vi "VI-Find Get Events Bottom.vi"(0 "VI in":refnum<vi>, 11 "error in (no error)":errorcluster) -> (4 "VI out":refnum<vi>, 6 "bundler":refnum<vi>, 10 "# of constants":i32, 13 "function pos":T1, 14 "constant pos":T1, 15 "error out":errorcluster)   [LabVIEW 2015]
uses:
  <vilib>/Utility/miscctls.llb/LVPointTypeDef.ctl
  <vilib>/Utility/traverseref.llb/TRef TravTarget.ctl
  <vilib>/Utility/traverseref.llb/VI Scripting - Traverse.lvlib
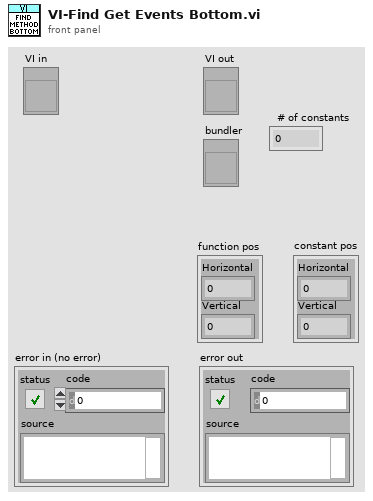
[diagram p1: front panel]
types:
  T1 = typedef "LVPointTypeDef.ctl" = cluster{"Horizontal":i16, "Vertical":i16}
  T2 = typedef "TRef TravTarget.ctl" = enum16{"FP", "BD", "Other"}
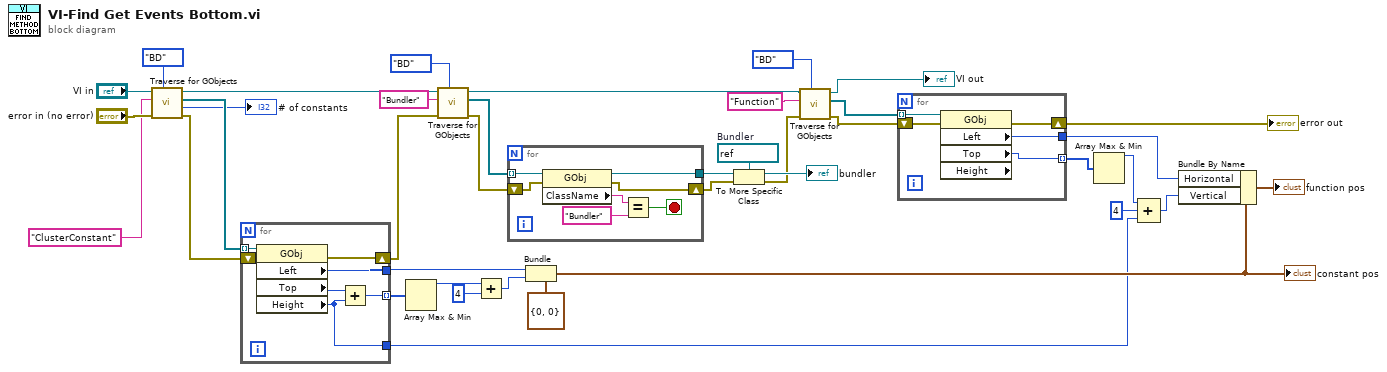
[diagram p0: block diagram]
diagram:
  w20 = refnum<vi> refnum  # Bundler
  n1 = call <vilib>:"Traverse for GObjects.vi"("Traverse Target"=TRef_TravTarget."BD", "error in (no error)"="error in (no error)", "Class Name"="ClusterConstant", "VI Refnum"="VI in") -> ("error out"=w28:errorcluster, "# of Refs"=→"# of constants":i32, "References"=w35:refnum<vi>[], "dup VI Refnum"=w27:refnum<vi>)  [unwired: 4 in]
  n2 = for {
    tunnel: w35 -> [w46] mode=indexing
    tunnel: [w45] -> w33
    tunnel: [w43] -> w34 mode=indexing
    shift-right: [w41] -> w26
    shift-left: w28 -> [w42]
    tunnel: [w40] -> w1
    n3 = property class="GObj"(reference=w46, error in=w42) -> (error out=w41:errorcluster, "Left"=w45:i32, "Top"=w44:i32, "Height"=w40:u32)  [unwired: 1 out]
    n4 = Add(x=w44, y=w40) -> (x+y=w43:u32)
  }
  n5 = Array Max & Min(array=w34) -> (max value=w32:u32)  [unwired: 3 out]
  n6 = call <vilib>:"Traverse for GObjects.vi"("Traverse Target"=TRef_TravTarget."BD", "error in (no error)"=w26, "Class Name"="Bundler", "VI Refnum"=w27) -> ("error out"=w16:errorcluster, "References"=w23:refnum<vi>[], "dup VI Refnum"=w15:refnum<vi>)  [unwired: 4 in, 1 out]
  n7 = Add(x=w32, y=u32 4) -> (x+y=w30:u32)
  n8 = for {
    tunnel: w23 -> [w53] mode=indexing
    shift-right: [w51] -> w21
    shift-left: w16 -> [w52]
    tunnel: [w50] -> w22
    stop <- w47 stop-if-true
    n9 = property class="GObj"(reference=w53, error in=w52) -> (reference out=w50:refnum<vi>, error out=w51:errorcluster, "ClassName"=w49:string)
    n10 = Equal?(x=w49, y="Bundler") -> (x = y?=w47:bool)
  }
  n11 = Bundle(cluster=T1 {"Horizontal"=0, "Vertical"=0} ("location"), "Horizontal"=w33, "Vertical"=w30) -> (w9:T1)
  "constant pos" <- w9
  n12 = To More Specific Class(target class=w20, reference=w22, error in=w21) -> (specific class reference=→"bundler":refnum<vi>, error out=w12:errorcluster)
  n13 = call <vilib>:"Traverse for GObjects.vi"("Traverse Target"=TRef_TravTarget."BD", "error in (no error)"=w12, "Class Name"="Function", "VI Refnum"=w15) -> ("error out"=w11:errorcluster, "References"=w6:refnum<vi>[], "dup VI Refnum"=→"VI out":refnum<vi>)  [unwired: 4 in, 1 out]
  n14 = for {
    tunnel: [w56] -> w8
    shift-right: [w57] -> w10
    shift-left: w11 -> [w58]
    tunnel: w6 -> [w55] mode=indexing
    tunnel: [w54] -> w5 mode=indexing
    n15 = property class="GObj" props=["Left", "Top", "Height"](reference=w55, error in=w58) -> (error out=w57:errorcluster, "Left"=w56:i32, "Top"=w54:i32)  [unwired: 2 out]
  }
  "error out" <- w10
  n16 = Array Max & Min(array=w5) -> (max value=w3:i32)  [unwired: 3 out]
  n17 = Compound Arithmetic op=ADD(w3, u32 4 ("y"), w1) -> (w2:u32)
  n18 = Bundle By Name(cluster=w9, "Horizontal"=w8, "Vertical"=w2) -> (→"function pos":T1)
